vi "Climb_Execute.vi"() -> ()   [LabVIEW 2019]
uses:
  Globals/Climb_Globals.vi
  <vilib>/Rock Robotics/WPI/Solenoid/WPI_SolenoidValue.ctl
  Globals/Solenoid Globals.vi
  <vilib>/Rock Robotics/WPI/Solenoid/WPI_SolenoidSetEnum.vi
panel:
  out "LeadScrew_Throttle":dbl
  out "Joint_Power":dbl
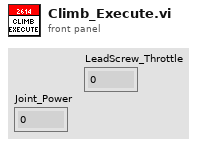
[diagram p1: front panel]
types:
  T1 = typedef "WPI_SolenoidDevRef.ctl" = cluster{"DevStatus":errorcluster, "Pneumatics Control Module":u8, "Forward Solenoid Channel":T2, "Reverse Solenoid Channel":T2}
  T2 = typedef "WPI_SolenoidChannel.ctl" = enum8{"Solenoid 0", "Solenoid 1", "Solenoid 2", "Solenoid 3", "Solenoid 4", "Solenoid 5", "Solenoid 6", "Solenoid 7", "Invalid"}
  T3 = typedef "WPI_SolenoidValue.ctl" = enum16{"Off", "On", "Forward", "Reverse"}
  T4 = typedef "Climb_Cluster.ctl" = cluster{"Control_State":T5, "Extend_Climber?":bool, "Clamp?":bool, "Balance?":bool, "Transverse_Throttle":dbl, "Elevator_Throttle":dbl, "Control_Panel_Setpoint?":bool, "Auto-Balance":bool, "Pivot_Throttle":dbl}
  T5 = typedef "Climb_States.ctl" = enum16{"No-Op", "Extending", "Clamping", "Balancing", "Manual_Control"}
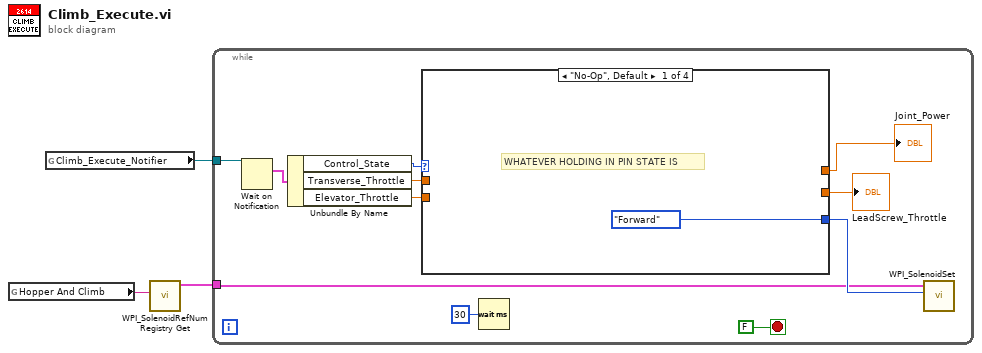
[diagram p0: block diagram]
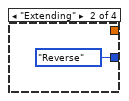
[diagram p2: hidden frame]
diagram:
  n1 = global read "Solenoid Globals.vi" "Hopper And Climb"() -> (w2:string)
  n2 = global read "Climb_Globals.vi" "Climb_Execute_Notifier"() -> (w3:refnum<notifier>)
  n3 = call <vilib>:"WPI_SolenoidRefNum Registry Get.vi"("refnum name"=w2) -> ("SolenoidDevRef"=w1:T1)  [unwired: 9 in, 1 out]
  n4 = while {
    tunnel: w3 -> [w13]
    tunnel: w1 -> [w4]
    stop <- FALSE stop-if-true
    n5 = Wait on Notification(notifier=w13) -> (notification=w12:T4)  [unwired: 3 in, 3 out]
    n6 = Unbundle By Name(w12) -> ("Control_State"=w11:T5, "Transverse_Throttle"=w10:dbl, "Elevator_Throttle"=w8:dbl)
    n7 = case shown="\"No-Op\", Default" w11 {
      tunnel: [WPI_SolenoidValue."Forward" ("Value") WPI_SolenoidValue."Reverse" ("Value") _ _] -> w5
      tunnel: w10 -> [_ _ _ w18]
      tunnel: [_ _ _ w18] -> w9
      tunnel: w8 -> [_ _ w17 _]
      tunnel: [_ _ w17 _] -> w7
      frame "No-Op", Default {
        # "WHATEVER HOLDING IN PIN STATE IS"
      }
      frame "Extending" {
      }
      frame "Clamping" {
        # "fully manual control atm"
      }
      frame "Balancing" {
        # "all manual right now, add in auto-balance"
      }
    }
    "Joint_Power" <- w9
    "LeadScrew_Throttle" <- w7
    n8 = Wait (ms)(milliseconds to wait=u32 30) -> ()  [unwired: 1 out]
    n9 = call-poly <vilib>:"WPI_SolenoidSet.vi"("Value"=w5, "SolenoidDevRef"=w4) -> ()  [unwired: 8 in, 2 out]
  }
